vi "3D Stack Prep.vi"() -> ()   [LabVIEW 2022 SP3]
uses:
  <vilib>/Utility/file.llb/Read From Spreadsheet File (DBL).vi
panel:
  out "Intensity Graph":u8[][](graph)
  out "size(s)":i32[](array[numeric])
  in  "pattern":string
  in  "Choose Directory":path
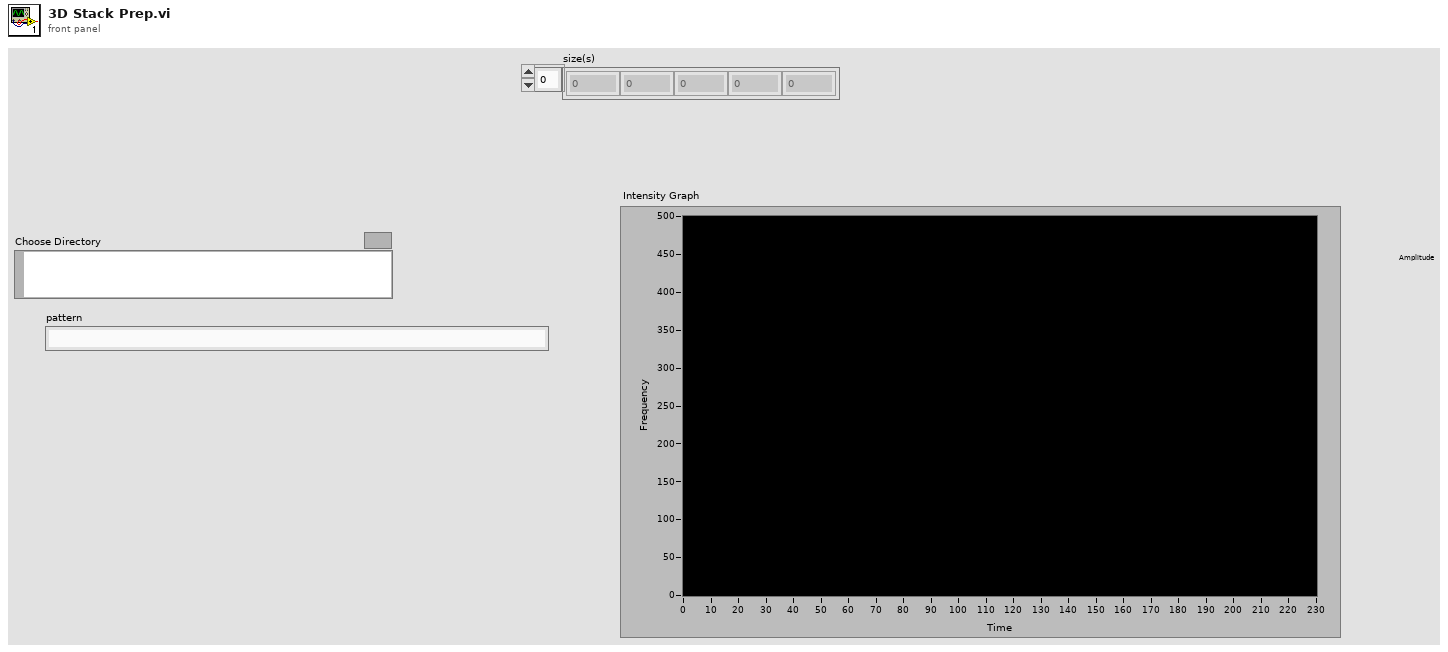
[diagram p1: front panel]
types:
  T1 = enum16{"open", "replace", "create", "open or create", "replace or create", "replace or create with confirmation"}
  T2 = enum16{"big-endian, network order", "native, host order", "little-endian"}
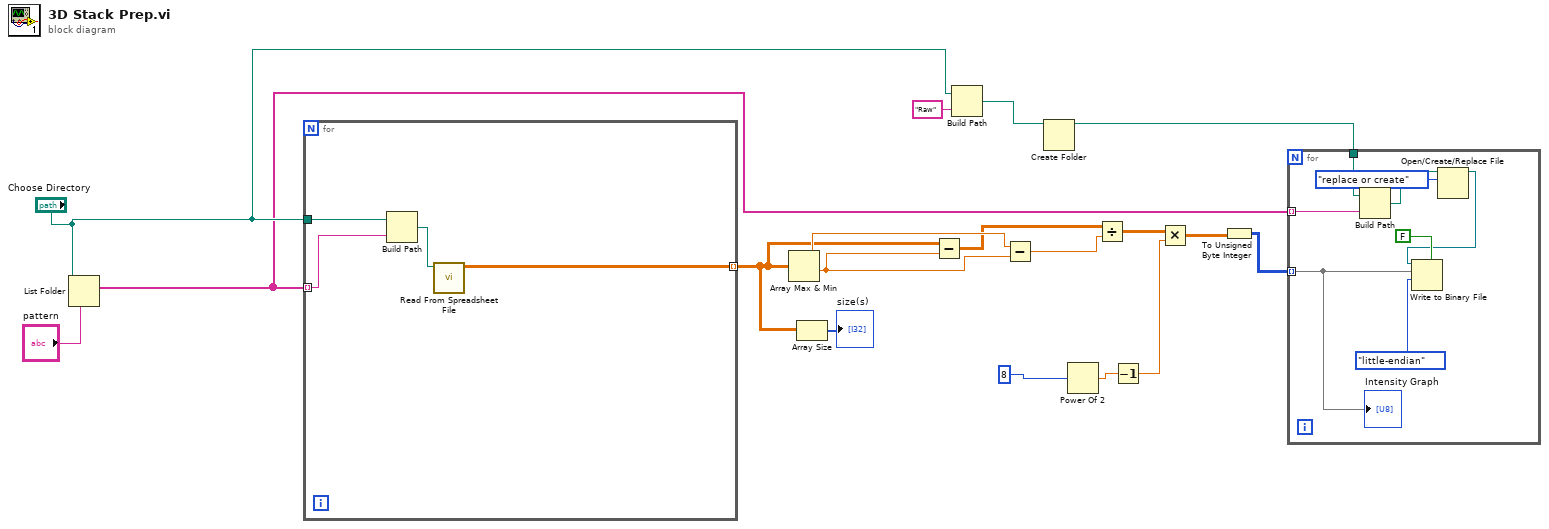
[diagram p0: block diagram]
diagram:
  n1 = List Folder(path="Choose Directory", pattern="pattern") -> (filenames=w5:string[])  [unwired: 1 in, 4 out]
  n2 = for {
    tunnel: w5 -> [w21] mode=indexing
    tunnel: "Choose Directory" -> [w22]
    tunnel: [w19] -> w2 mode=indexing
    n3 = Build Path(base path=w22, name or relative path=w21) -> (appended path=w20:path)
    n4 = call-poly <vilib>:"Read From Spreadsheet File.vi"("file path (dialog if empty)"=w20) -> ("all rows"=w19:dbl[][])  [unwired: 6 in, 4 out]
  }
  n5 = Array Max & Min(array=w2) -> (max value=w16:dbl, min value=w17:dbl)  [unwired: 2 out]
  n6 = Array Size(array=w2) -> (size(s)=→"size(s)":i32[])
  n7 = Subtract(x=w2, y=w17) -> (x-y=w14:dbl[][][])
  n8 = Build Path(base path="Choose Directory", name or relative path="Raw") -> (appended path=w4:path)
  n9 = Subtract(x=w16, y=w17) -> (x-y=w15:dbl)
  n10 = Create Folder(path (use dialog)=w4) -> (created path=w3:path)  [unwired: 2 in, 2 out]
  n11 = Power Of 2(x=8) -> (2^x=w11:dbl)
  n12 = Divide(x=w14, y=w15) -> (x/y=w13:dbl[][][])
  n13 = Decrement(x=w11) -> (x-1=w10:dbl)
  n14 = Multiply(x=w13, y=w10) -> (x*y=w7:dbl[][][])
  n15 = To Unsigned Byte Integer(number=w7) -> (unsigned 8bit integer=w6:u8[][][])
  n16 = for {
    tunnel: w6 -> [w23] mode=indexing
    tunnel: w5 -> [w30] mode=indexing
    tunnel: w3 -> [w29]
    n17 = Build Path(base path=w29, name or relative path=w30) -> (appended path=w26:path)
    n18 = Open/Create/Replace File(file path (use dialog)=w26, operation (0:open)=T1."replace or create") -> (refnum out=w25:refnum<file>)  [unwired: 4 in, 2 out]
    n19 = Write to Binary File(file (use dialog)=w25, data=w23, 5:FALSE ("prepend array or string size? (T)"), 9:T2."little-endian" ("byte order (0:big-endian, network order)")) -> ()  [unwired: 2 in, 3 out]
    "Intensity Graph" <- w23
  }
